vi "Add Sections.vi"(8 "error in (no error)":errorcluster, 11 "Item Ref in":T1 format="%.0x") -> (0 "error out":errorcluster, 3 "Item Ref out":T1 format="%.0x")   [LabVIEW 2019, in "Profile Interpolation System Explorer.lvlib"]
uses:
  Profile Interpolation System Explorer.lvlib
  <vilib>/NI VeriStand/Custom Device API/Custom Device API.lvlib
  Shared/SubVIs/Constants.vi
  Shared/Profile Interpolation Shared.lvlib
  <vilib>/NI VeriStand/Custom Device API/Custom Device Item Ref.ctl
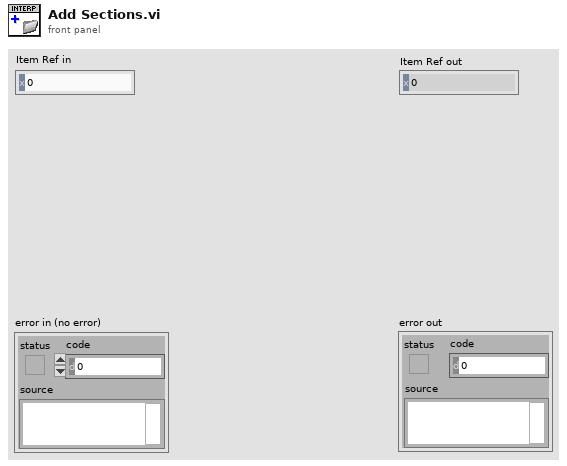
[diagram p1: front panel]
types:
  T1 = typedef "Custom Device API.lvlib/Custom Device Item Ref.ctl" = u64
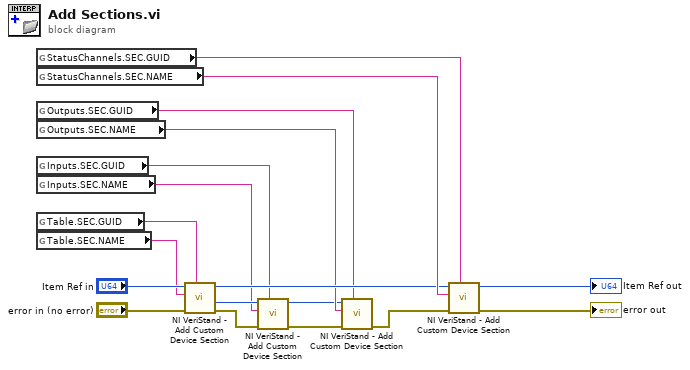
[diagram p0: block diagram]
diagram:
  n1 = global read "Constants.vi" "StatusChannels.SEC.GUID"() -> (w17:string)
  n2 = global read "Constants.vi" "StatusChannels.SEC.NAME"() -> (w14:string)
  n3 = global read "Constants.vi" "Outputs.SEC.GUID"() -> (w5:string)
  n4 = global read "Constants.vi" "Outputs.SEC.NAME"() -> (w4:string)
  n5 = global read "Constants.vi" "Inputs.SEC.GUID"() -> (w8:string)
  n6 = global read "Constants.vi" "Inputs.SEC.NAME"() -> (w7:string)
  n7 = global read "Constants.vi" "Table.SEC.GUID"() -> (w13:string)
  n8 = global read "Constants.vi" "Table.SEC.NAME"() -> (w12:string)
  n9 = call <vilib>:"NI VeriStand - Add Custom Device Section.vi"("GUID (Default Section)"=w13, "error in (no error)"="error in (no error)", "Section Name"=w12, "Parent Ref in"="Item Ref in") -> ("error out"=w10:errorcluster, "Section Ptr"=w9:T1, "Parent Ref out"=w11:T1)  [unwired: 4 in, 1 out]
  n10 = call <vilib>:"NI VeriStand - Add Custom Device Section.vi"("GUID (Default Section)"=w8, "error in (no error)"=w10, "Section Name"=w7, "Parent Ref in"=w9) -> ("error out"=w1:errorcluster, "Parent Ref out"=w2:T1)  [unwired: 4 in, 2 out]
  n11 = call <vilib>:"NI VeriStand - Add Custom Device Section.vi"("GUID (Default Section)"=w5, "error in (no error)"=w1, "Section Name"=w4, "Parent Ref in"=w2) -> ("error out"=→"error out":errorcluster)  [unwired: 4 in, 3 out]
  n12 = call <vilib>:"NI VeriStand - Add Custom Device Section.vi"("GUID (Default Section)"=w17, "Section Name"=w14, "Parent Ref in"=w11) -> ("Parent Ref out"=→"Item Ref out":T1)  [unwired: 5 in, 3 out]
